vi "Puff_realisation_display.vi"(2 "Actual Sampling rate (Hz)":dbl=1000.0 format="%.2f", 3 "Input Array":dbl[](array[numeric]) format="%.2f") -> ()   [LabVIEW 2010]
panel:
  in  "Case Constant\n(See Context Help)":bool=TRUE
  out "Puff Trace":cluster{dbl, dbl, dbl[]}[](graph)
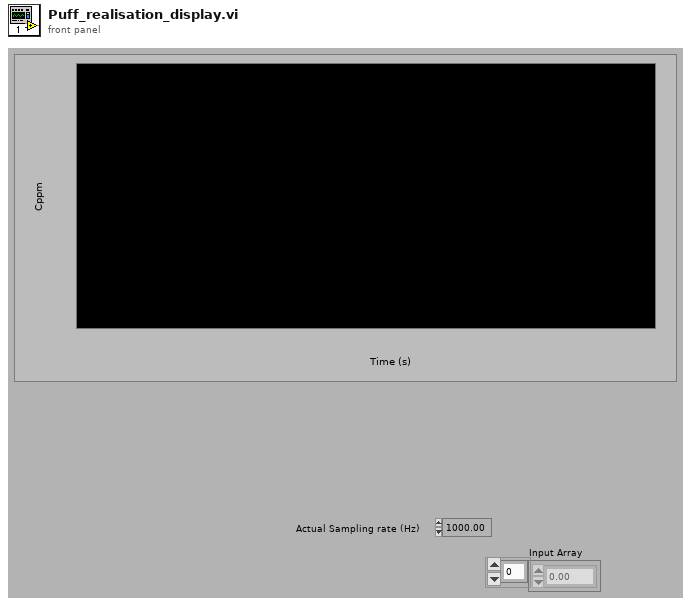
[diagram p1: front panel]
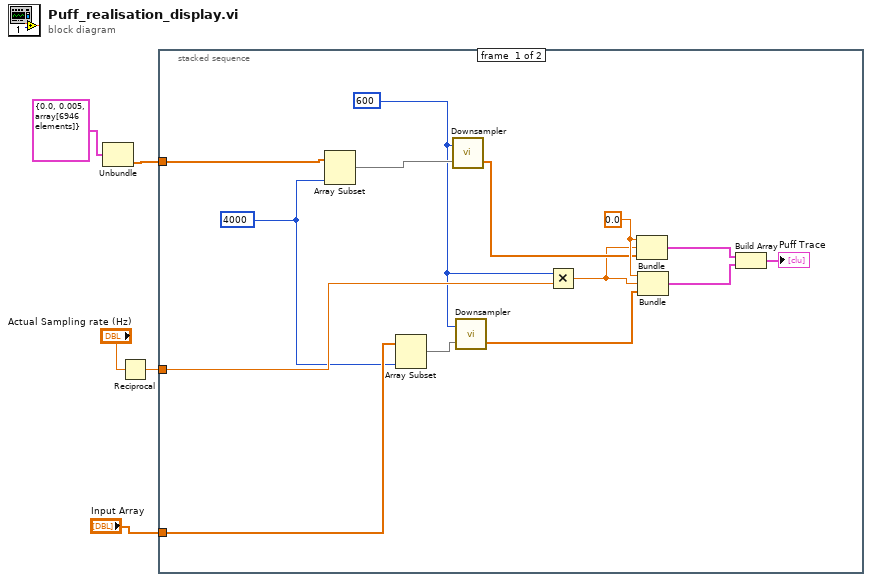
[diagram p0: block diagram]
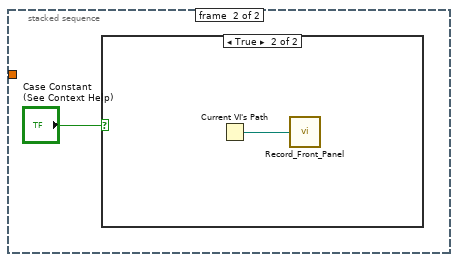
[diagram p2: hidden frame]
diagram:
  n1 = Unbundle(cluster{dbl, dbl, dbl[]} {0.0, 0.005, array[6946 elements]} ("FFID Trace")) -> (w5:dbl[])  [unwired: 2 out]
  n2 = Reciprocal(x="Actual Sampling rate (Hz)") -> (1/x=w2:dbl)
  n3 = stacked-sequence {
    tunnel: w5 -> [w11 _]
    tunnel: "Input Array" -> [w9 _]
    tunnel: w2 -> [w16 _]
    frame #0 {
      w7 = 4000 ("Array length")
      w6 = 600 ("Averaging samples")
      w19 = 0.0
      n4 = Array Subset(array=w11, length=w7) -> (w10:dbl[])  [unwired: 1 in]
      n5 = Array Subset(array=w9, length=w7) -> (w8:dbl[])  [unwired: 1 in]
      n6 = call "Downsampler.vi"("Input Array"=w10, "Averaging samples"=w6) -> ("Downsampled Array"=w17:dbl[])  [unwired: 1 out]
      n7 = call "Downsampler.vi"("Input Array"=w8, "Averaging samples"=w6) -> ("Downsampled Array"=w18:dbl[])  [unwired: 1 out]
      n8 = Multiply(x=w6, y=w16) -> (x*y=w15:dbl)
      n9 = Bundle(w19, w15, "Downsampled Array"=w17) -> (w13:cluster{dbl, dbl, "Downsampled Array":dbl[]})  [unwired: 1 out]
      n10 = Bundle(w19, w15, "Downsampled Array"=w18) -> (w14:cluster{dbl, dbl, "Downsampled Array":dbl[]})  [unwired: 1 out]
      n11 = Build Array(w13, w14) -> (→"Puff Trace":cluster{dbl, dbl, "Downsampled Array":dbl[]}[])
    }
    frame #1 {
      n12 = case shown="True" "Case Constant\n(See Context Help)" {
        frame False {
        }
        frame True {
          n13 = Current VI's Path() -> (path=w21:path)
          n14 = call "Record_Front_Panel.vi"("VI to Log"=w21) -> ()  [unwired: 1 out]
        }
      }
    }
  }
